vi "Cache Resource Info.vi"(8 "error in (no error)":errorcluster, 11 "Session in":refnum<class "Session.lvclass">) -> (0 "error out":errorcluster, 3 "Session out":refnum<class "Session.lvclass">)   [LabVIEW 2024, in "CTI.lvlib" / "Session.lvclass"]
uses:
  Session.lvclass
  Session.lvclass/Session.ctl
  2901766c-f06d-4bd9-a239-148df5fac322.vi
  Is Full Errors.vi
  Check Errors.vi
  DeviceComms/DeviceComms.lvclass
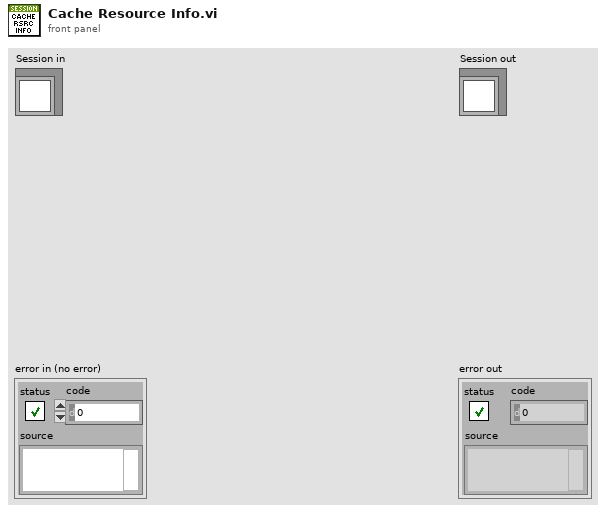
[diagram p1: front panel]
types:
  T1 = typedef "CTI.lvlib/GPIO Number.ctl" = i8
  T2 = typedef "CTI.lvlib/Available AI.ctl" = cluster{"ADC #":T3, "GPIO #":T1}
  T3 = typedef "CTI.lvlib/ADC Number.ctl" = i8
  T4 = typedef "CTI.lvlib/Available UART.ctl" = cluster{"UART #":T5, "TX GPIOs":T1[], "RX GPIOs":T1[]}
  T5 = typedef "CTI.lvlib/UART Number.ctl" = i8
  T6 = typedef "CTI.lvlib/Available I2C.ctl" = cluster{"I2C #":T7, "SCL GPIOs":T1[], "SDA GPIOs":T1[]}
  T7 = typedef "CTI.lvlib/I2C Number.ctl" = i8
  T8 = typedef "CTI.lvlib/Available SPI.ctl" = cluster{"SPI #":T9, "TX GPIOs":T1[], "RX GPIOs":T1[], "SCK GPIOs":T1[]}
  T9 = typedef "CTI.lvlib/SPI Number.ctl" = i8
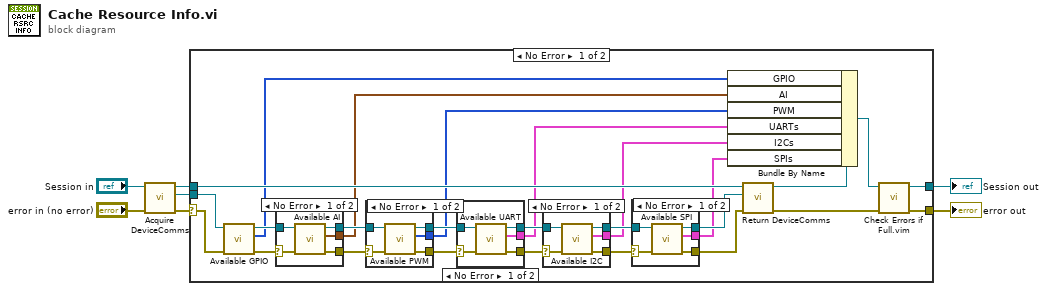
[diagram p0: block diagram]
diagram:
  n1 = call "Acquire DeviceComms.vi"("error in (no error)"="error in (no error)", "Session in"="Session in") -> ("error out"=w5:errorcluster, "DeviceComms"=w4:refnum<class "DeviceComms.lvclass">, "Session out"=w3:refnum<class "Session.lvclass">)  [unwired: 7 in]
  n2 = case shown="No Error" w5 {
    selector: w5 -> [w32 w69]
    tunnel: w4 -> [w33 _]
    tunnel: w3 -> [w29 w70]
    tunnel: [w9 w69] -> w2
    tunnel: [w8 w70] -> w1
    frame No Error {
      n3 = call-dynamic "Available GPIO.vi"("error in (no error)"=w32, "DeviceComms in"=w33) -> ("error out"=w30:errorcluster, "Available GPIO"=w28:T1[], "DeviceComms out"=w31:refnum<class "DeviceComms.lvclass">)  [unwired: 7 in]
      n4 = case shown="No Error" w30 {
        selector: w30 -> [w37 w39]
        tunnel: w31 -> [w38 w40]
        tunnel: [w36 w40] -> w27
        tunnel: [w35 w39] -> w26
        tunnel: [w34 _] -> w25
        frame No Error {
          n5 = call-dynamic "Available AI.vi"("error in (no error)"=w37, "DeviceComms in"=w38) -> ("error out"=w35:errorcluster, "Available AI"=w34:T2[], "DeviceComms out"=w36:refnum<class "DeviceComms.lvclass">)  [unwired: 7 in]
        }
        frame Error {
        }
      }
      n6 = case shown="No Error" w26 {
        selector: w26 -> [w44 w46]
        tunnel: w27 -> [w45 w47]
        tunnel: [w43 w47] -> w24
        tunnel: [w42 w46] -> w23
        tunnel: [w41 _] -> w18
        frame No Error {
          n7 = call-dynamic "Available PWM.vi"("error in (no error)"=w44, "DeviceComms in"=w45) -> ("error out"=w42:errorcluster, "Available PWM"=w41:T1[], "DeviceComms out"=w43:refnum<class "DeviceComms.lvclass">)  [unwired: 7 in]
        }
        frame Error {
        }
      }
      n8 = case shown="No Error" w23 {
        selector: w23 -> [w51 w53]
        tunnel: w24 -> [w52 w54]
        tunnel: [w50 w54] -> w22
        tunnel: [w49 w53] -> w21
        tunnel: [w48 _] -> w17
        frame No Error {
          n9 = call-dynamic "Available UART.vi"("error in (no error)"=w51, "DeviceComms in"=w52) -> ("error out"=w49:errorcluster, "Available UART"=w48:T4[], "DeviceComms out"=w50:refnum<class "DeviceComms.lvclass">)  [unwired: 7 in]
        }
        frame Error {
        }
      }
      n10 = case shown="No Error" w21 {
        selector: w21 -> [w58 w60]
        tunnel: w22 -> [w59 w61]
        tunnel: [w57 w61] -> w20
        tunnel: [w56 w60] -> w19
        tunnel: [w55 _] -> w16
        frame No Error {
          n11 = call-dynamic "Available I2C.vi"("error in (no error)"=w58, "DeviceComms in"=w59) -> ("error out"=w56:errorcluster, "Available I2C"=w55:T6[], "DeviceComms out"=w57:refnum<class "DeviceComms.lvclass">)  [unwired: 7 in]
        }
        frame Error {
        }
      }
      n12 = case shown="No Error" w19 {
        selector: w19 -> [w65 w67]
        tunnel: w20 -> [w66 w68]
        tunnel: [w64 w68] -> w14
        tunnel: [w63 w67] -> w13
        tunnel: [w62 _] -> w12
        frame No Error {
          n13 = call-dynamic "Available SPI.vi"("error in (no error)"=w65, "DeviceComms in"=w66) -> ("error out"=w63:errorcluster, "Available SPI"=w62:T8[], "DeviceComms out"=w64:refnum<class "DeviceComms.lvclass">)  [unwired: 7 in]
        }
        frame Error {
        }
      }
      n14 = call "Return DeviceComms.vi"("error in (no error)"=w13, "DeviceComms"=w14, "Session in"=w29) -> ("error out"=w10:errorcluster, "Session out"=w15:refnum<class "Session.lvclass">)  [unwired: 7 in]
      n15 = Bundle By Name(cluster=w15, "GPIO"=w28, "AI"=w25, "PWM"=w18, "UARTs"=w17, "I2Cs"=w16, "SPIs"=w12) -> (w11:refnum<class "Session.lvclass">)
      n16 = call "Check Errors if Full.vim"("error in (no error)"=w10, "Session in"=w11) -> ("error out"=w9:errorcluster, "Session out"=w8:refnum<class "Session.lvclass">)  [unwired: 8 in]
    }
    frame Error {
    }
  }
  "error out" <- w2
  "Session out" <- w1
